vi "sub_Get Error Log Path.vi"(8 "error in (no error)":errorcluster) -> (0 "error out":errorcluster, 3 "Path":path)   [LabVIEW 2016, in "System.lvlib"]
uses:
  System.lvlib
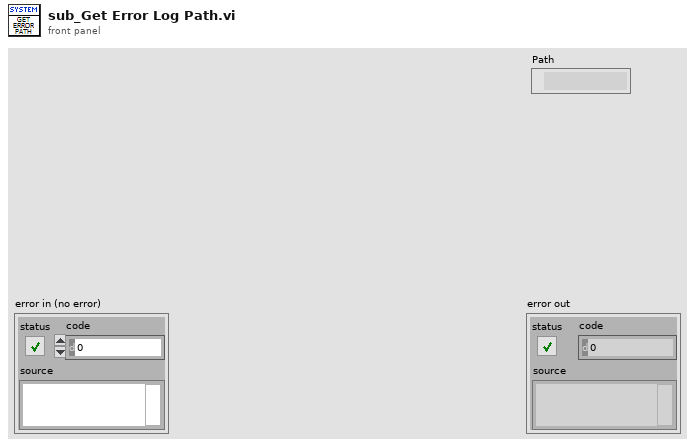
[diagram p1: front panel]
types:
  T1 = typedef "System.lvlib/Control_Variant Data Reference.ctl" = refnum<data-value>
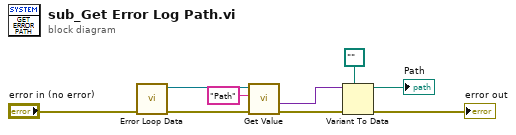
[diagram p0: block diagram]
diagram:
  n1 = call "Error Loop Data.vi"("error in (no error)"="error in (no error)") -> ("error out"=w8:errorcluster, "Error Data Reference"=w7:T1)  [unwired: 9 in]
  n2 = call "Get Value.vi"("error in (no error)"=w8, "Name"="Path", "Data Reference"=w7) -> ("error out"=w5:errorcluster, "Value"=w4:variant)  [unwired: 7 in]
  n3 = Variant To Data(error in=w5, type=path "", Variant=w4) -> (data=→"Path":path, error out=→"error out":errorcluster)
